vi "Drum.vi"() -> ()   [LabVIEW 2012]
uses:
  <vilib>/ptbypt/NI_PtbyPt.lvlib
panel:
  in  "alpha":dbl(slide) scale=0.0..10.0
  in  "stop":bool
  in  "P":i32(slide) scale=0.0..10.0
  out "Waveform Graph":waveform(dbl)(graph)
  in  "N":i32(slide) scale=0.0..10.0
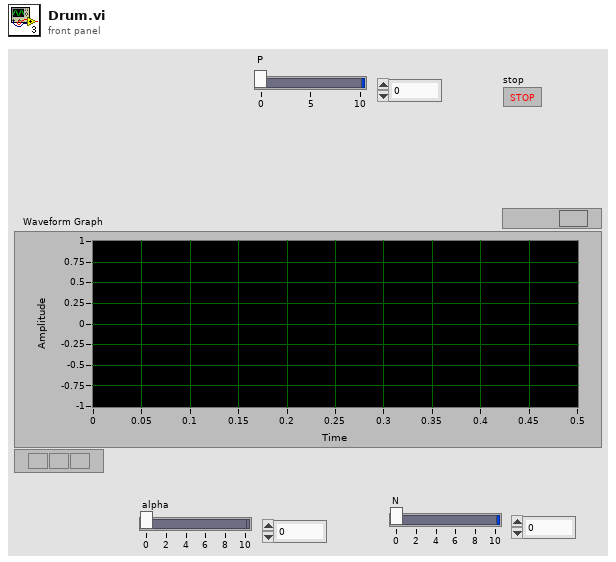
[diagram p1: front panel]
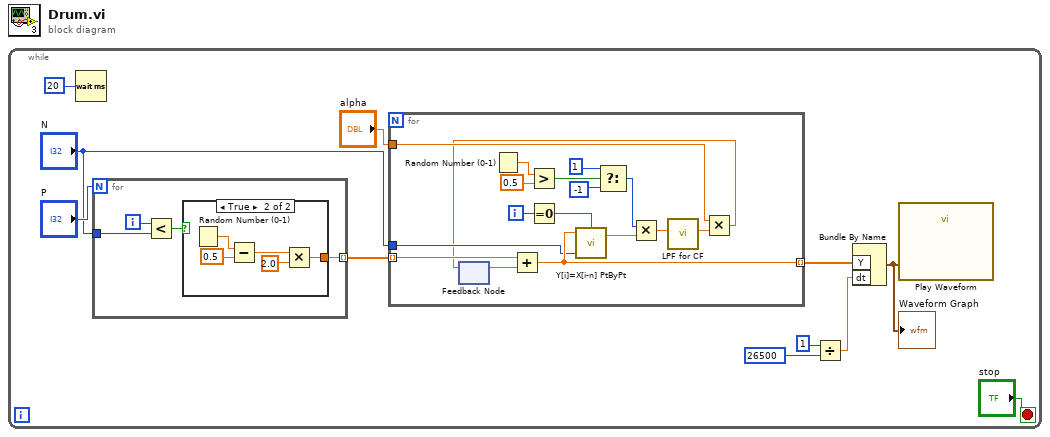
[diagram p0: block diagram]
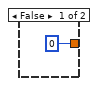
[diagram p2: hidden frame]
diagram:
  n1 = while {
    stop <- "stop" stop-if-true
    n2 = Wait (ms)(milliseconds to wait=20) -> ()  [unwired: 1 out]
    n3 = for {
      N: "P" -> [_]
      tunnel: [w32] -> w4 mode=indexing
      tunnel: "N" -> [w29]
      i -> [w30]
      n4 = Less?(x=w30, y=w29) -> (x < y?=w31:bool)
      n5 = case shown="True" w31 {
        tunnel: [0 w36] -> w32
        frame False {
        }
        frame True {
          n6 = Random Number (0-1)() -> (number: 0 to 1=w38:dbl)
          n7 = Subtract(x=w38, y=0.5) -> (x-y=w35:dbl)
          n8 = Multiply(x=w35, y=2.0) -> (x*y=w36:dbl)
        }
      }
    }
    n9 = for {
      tunnel: w4 -> [w21] mode=indexing
      tunnel: "N" -> [w14]
      tunnel: "alpha" -> [w20]
      tunnel: [w16] -> w2 mode=indexing
      i -> [w22]
      n10 = feedback #1() -> (w12:dbl)  [unwired: 1 in]
      n11 = Random Number (0-1)() -> (number: 0 to 1=w27:dbl)
      n12 = Add(x=w21, y=w12) -> (x+y=w16:dbl)
      n13 = Greater?(x=w27, y=0.5) -> (0:w26:bool)
      n14 = Equal To 0?(x=w22) -> (x = 0?=w23:bool)
      n15 = call <vilib>:"Y[i]=X[i-n] PtByPt.vi"("initialize"=w23, "shifts: n"=w14, "x"=w16) -> ("shifted x"=w15:dbl)  [unwired: 1 in, 1 out]
      n16 = Select(t=1, s=w26, f=-1) -> (s? t:f=w18:i32)
      n17 = Multiply(x=w18, y=w15) -> (x*y=w17:dbl)
      n18 = call "LPF for CF.vi"("Numeric"=w17) -> ("Numeric 2"=w19:dbl)  [unwired: 10 in]
      n19 = Multiply(x=w20, y=w19) -> (x*y=w13:dbl)
      n20 = feedback-in #1(w13) -> ()
    }
    n21 = Divide(x=1, y=26500) -> (x/y=w7:dbl)
    n22 = Bundle By Name("Y"=w2, "dt"=w7) -> (w10:waveform(dbl))  [unwired: 1 in]
    "Waveform Graph" <- w10
    n23 = call "Play Waveform"("Data"=w10) -> ()  [unwired: 18 in, 1 out]
  }
